vi "Drop Message Core.vi"(11 "Response Msg in":refnum<class "Response Msg.lvclass">) -> ()   [LabVIEW 2020, in "Publisher.lvlib" / "Response Msg.lvclass"]
doc: "(<B>Filename</B>: Actor Framework.lvlib:Message.lvclass:Drop Message Core.vi)\n\nDefines what a message does if it is in the message queue when the queue is released. At this point, the actor has shut down, so it will never process the message.\n\nCall parent method and call the Drop method on the Response Core."
uses:
  Response Msg.lvclass
  Response Msg.lvclass/Response Msg.ctl
  Response Core/Response Core/Response Core.lvclass
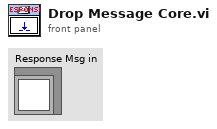
[diagram p1: front panel]
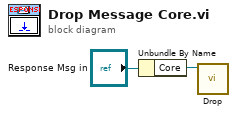
[diagram p0: block diagram]
diagram:
  n1 = Unbundle By Name("Response Msg in") -> ("Core"=w1:refnum<class "Response Core.lvclass">)
  n2 = call-dynamic "Drop.vi"("Response Core in"=w1) -> ()  [unwired: 11 in]
